vi "util_transition_automatic.vi"(7 "transition_queue":refnum<queue>, 8 "error in (no error)":errorcluster, 10 "data":variant, 11 "recipe_data":variant) -> (0 "error out":errorcluster)   [LabVIEW 2015, in "lv-recipe-machine.lvlib"]
uses:
  lv-recipe-machine.lvlib
  _controls/transition.ctl
  _controls/change.ctl
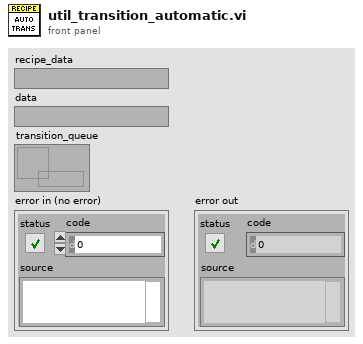
[diagram p1: front panel]
types:
  T1 = cluster{"change_in_event":refnum<user-event>, "transition_queue":refnum<queue>}
  T2 = cluster{"change_in_event":bool, "transition_queue":bool}
  T3 = typedef "lv-recipe-machine.lvlib/references.ctl" = cluster{"semaphore":T4, "input_queue":refnum<queue>, "output_queue":refnum<queue>, "transition_queue":refnum<queue>, "data_dvr":refnum<data-value>, "stop_notifier":refnum<notifier>, "change_in_event":refnum<user-event>, "change_out_event":refnum<user-event>, "status_event":refnum<user-event>}
  T4 = typedef "Semaphore RefNum" = refnum<k1>
  T5 = typedef "lv-recipe-machine.lvlib/transition.ctl" = cluster{"next_index":i32, "data":variant, "recipe_data":variant, "error":errorcluster}
  T6 = typedef "lv-recipe-machine.lvlib/change.ctl" = cluster{"data":variant}
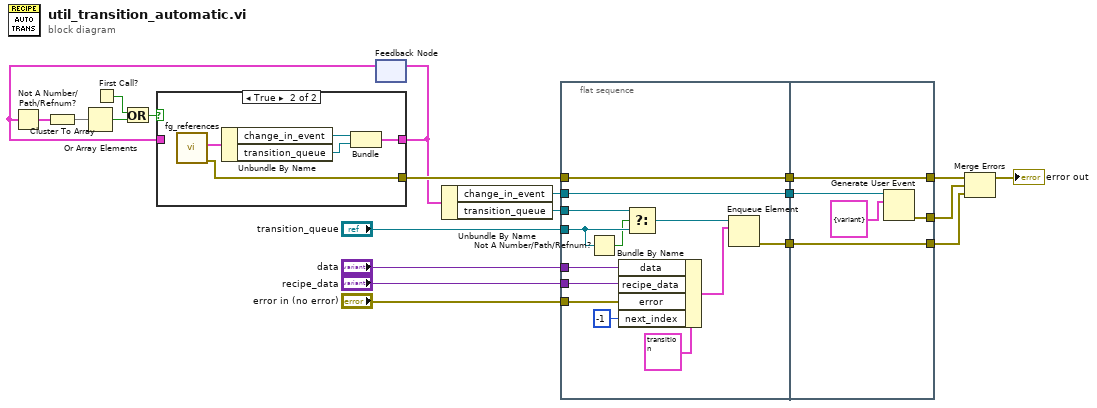
[diagram p0: block diagram]
diagram:
  n1 = First Call?() -> (First Call?: T/F=w11:bool)
  n2 = feedback #1() -> (w10:T1)  [unwired: 1 in]
  n3 = Not A Number/Path/Refnum?(number/path/refnum=w10) -> (NaN/Path/Refnum?=w12:T2)
  n4 = Cluster To Array(cluster=w12) -> (array=w8:bool[])
  n5 = Or Array Elements(Boolean array=w8) -> (logical OR=w7:bool)
  n6 = Or(x=w11, y=w7) -> (x .or. y?=w9:bool)
  n7 = case shown="True" w9 {
    tunnel: [_ w27] -> w21
    tunnel: [w22 w24] -> w6
    tunnel: w10 -> [w22 _]
    frame False {
    }
    frame True {
      n8 = call "fg_references.vi"() -> ("error out"=w27:errorcluster, "references out"=w26:T3)  [unwired: 10 in]
      n9 = Unbundle By Name(w26) -> ("change_in_event"=w25:refnum<user-event>, "transition_queue"=w23:refnum<queue>)
      n10 = Bundle("change_in_event"=w25, "transition_queue"=w23) -> (w24:T1)  [unwired: 1 in]
    }
  }
  n11 = feedback-in #1(w6) -> ()
  n12 = Unbundle By Name(w6) -> ("change_in_event"=w4:refnum<user-event>, "transition_queue"=w5:refnum<queue>)
  n13 = flat-sequence {
    tunnel: w4 -> [w40]
    tunnel: [w40] -> w18
    tunnel: w5 -> [w31]
    tunnel: "data" -> [w36]
    tunnel: "recipe_data" -> [w35]
    tunnel: "error in (no error)" -> [w34]
    tunnel: [w33] -> w14
    tunnel: w21 -> [w32]
    tunnel: [w32] -> w3
    tunnel: "transition_queue" -> [w29]
    tunnel: [w44] -> w20
    tunnel: w18 -> [w43]
    tunnel: w14 -> [w45]
    tunnel: [w45] -> w13
    tunnel: w3 -> [w41]
    tunnel: [w41] -> w2
    frame #0 {
      n14 = Not A Number/Path/Refnum?(number/path/refnum=w29) -> (NaN/Path/Refnum?=w28:bool)
      n15 = Bundle By Name(cluster=T5 {"next_index"=0, "data"=variant, "recipe_data"=variant, "error"={"status"=FALSE, "code"=0, "source"=""}} ("transition"), "data"=w36, "recipe_data"=w35, "error"=w34, "next_index"=-1) -> (w37:T5)
      n16 = Select(t=w31, s=w28, f=w29) -> (s? t:f=w30:refnum<queue>)
      n17 = Enqueue Element(queue=w30, element=w37) -> (error out=w33:errorcluster)  [unwired: 2 in, 2 out]
    }
    frame #1 {
      n18 = Generate User Event(user event=w43, event data cluster=T6 {"data"=variant} ("change")) -> (error out=w44:errorcluster)  [unwired: 2 in, 1 out]
    }
  }
  n19 = Merge Errors(w2, w20, w13) -> (→"error out":errorcluster)
